vi "GT Get Capture Home Gpi.vi"(0 "cardNum":i16, 1 "pGpiSts":i16, 2 "count":i16, 5 "trigger":i16, 7 "pHomeSts":i16, 9 "pHomePos":i16, 11 "error in (no error)":errorcluster caption="错误输入（无错误）", 12 "pGpiPos":i16) -> (4 "function return":i16, 10 "pHomePos out":i16, 14 "pGpiPos out":i16, 15 "error out":errorcluster caption="错误输出")   [LabVIEW 2020, in "gts.lvlib"]
doc: "GT_API GT_GetCaptureHomeGpi(short cardNum,short trigger,short pHomeSts,short *pHomePos,short pGpiSts,short *pGpiPos,short count=1);"
uses:
  gts.lvlib
  dll/32bit/multi_card/gts.dll
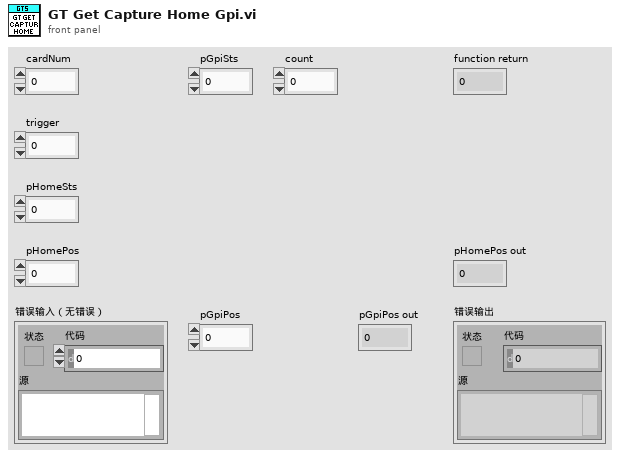
[diagram p1: front panel]
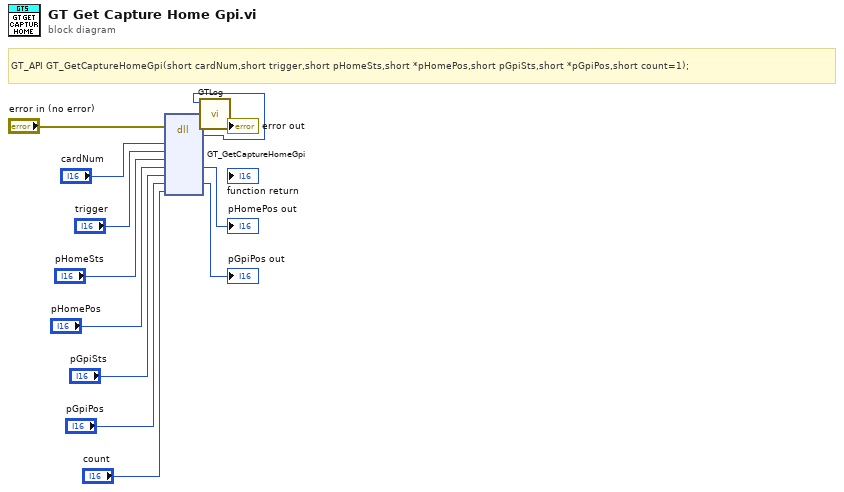
[diagram p0: block diagram]
diagram:
  # "GT_API GT_GetCaptureHomeGpi(short cardNum,short trigger,short pHomeSts,short *pHomePos,short pGpiSts,short *pGpiPos,short count=1);"
  n1 = dll-call lib="C:/1228/dll/32bit/multi_card/gts.dll" fn="GT_GetCaptureHomeGpi"(error in="error in (no error)", "cardNum"="cardNum", "trigger"="trigger", "pHomeSts"="pHomeSts", "pHomePos"="pHomePos", "pGpiSts"="pGpiSts", "pGpiPos"="pGpiPos", "count"="count") -> (error out=w3:errorcluster, w1:i16, "pHomePos"=→"pHomePos out":i16, "pGpiPos"=→"pGpiPos out":i16)  [unwired: 7 in, 1 out]
  n2 = call "GTLog.vi"("error in (no error)"=w3, "Numeric"=w1) -> ("error out"=→"error out":errorcluster)  [unwired: 9 in]
